vi "DelaySystem.vi"(8 "error in (no error)":errorcluster caption="错误输入（无错误）", 9 "system":dbl, 10 "delay":dbl, 11 "Path":path) -> (0 "error out":errorcluster caption="错误输出", 3 "delaySystem":u8)   [LabVIEW 2015]
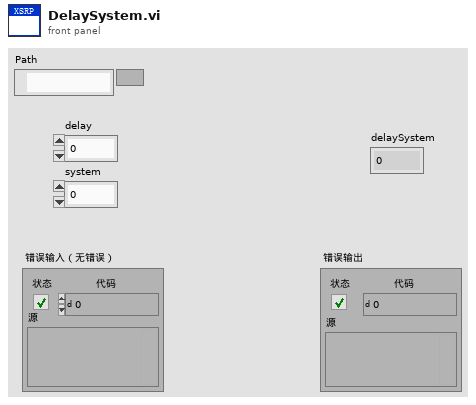
[diagram p1: front panel]
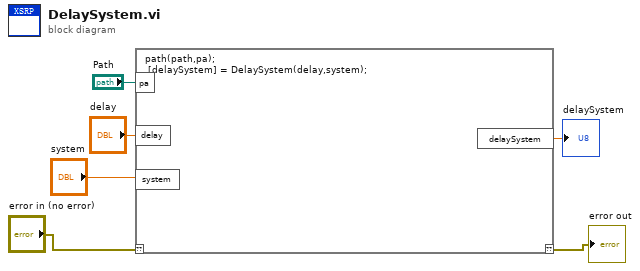
[diagram p0: block diagram]
diagram:
  n1 = script code="path(path,pa);\n [delaySystem] = DelaySystem(delay,system);"("??"="error in (no error)", "pa"="Path", "delay"="delay", "system"="system") -> ("??"=→"error out":errorcluster, "delaySystem"=→"delaySystem":dbl)
